vi "AE User Events.vi"(7 "Action":T1, 8 "error in (no error)":errorcluster, 10 "User Event":string, 11 "user event in":refnum<user-event>) -> (0 "error out":errorcluster, 3 "user event out":refnum<user-event>)   [LabVIEW 2013, in "main.lvlib"]
uses:
  main.lvlib
  Controls/Enum User Events.ctl
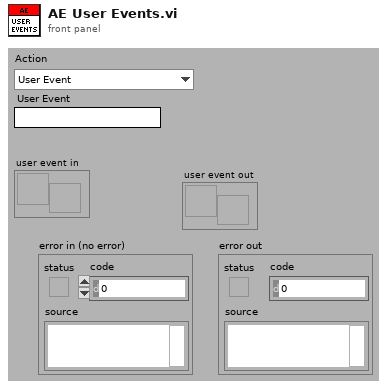
[diagram p1: front panel]
types:
  T1 = typedef "main.lvlib/Enum User Events.ctl" = enum16{"User Event", "Init"}
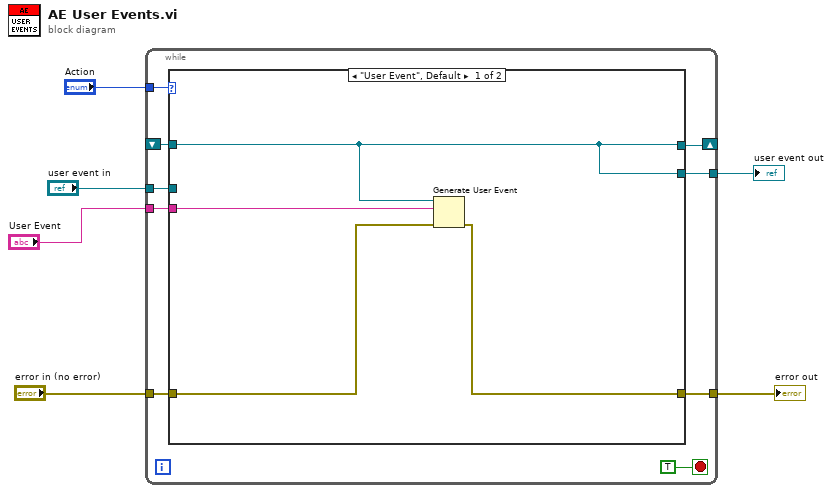
[diagram p0: block diagram]
diagram:
  n1 = while {
    shift-right: [w13] -> _
    shift-left: _ -> [w12]
    tunnel: "Action" -> [w15]
    tunnel: "user event in" -> [w14]
    tunnel: [w11] -> w4
    tunnel: "User Event" -> [w9]
    tunnel: "error in (no error)" -> [w8]
    tunnel: [w7] -> w1
    stop <- TRUE stop-if-true
    n2 = case shown="\"User Event\", Default" w15 {
      tunnel: [w19 w21] -> w13
      tunnel: w14 -> [_ w21]
      tunnel: w12 -> [w19 _]
      tunnel: [w19 w21] -> w11
      tunnel: w9 -> [w18 _]
      tunnel: w8 -> [w17 w20]
      tunnel: [w16 w20] -> w7
      frame "User Event", Default {
        n3 = Generate User Event(user event=w19, event data cluster=w18, error in=w17) -> (error out=w16:errorcluster)  [unwired: 1 in, 1 out]
      }
      frame "Init" {
      }
    }
  }
  "user event out" <- w4
  "error out" <- w1
